vi "Example_Simple Write and Read.vi"() -> ()   [LabVIEW 2018]
uses:
  Types/TCP Config_Cluster.ctl
  MB PLC Client.lvclass
  Types/PLC Config_Cluster.ctl
  Types/MB Ref Range_Cluster.ctl
  Types/Serial Config_Cluster.ctl
  MB PLC Client.lvclass/MB PLC Client.ctl
  791ddaad-21aa-49d1-827f-859499192ae9.vi
  2a8f512b-755f-4b06-8394-ae6f99e928d5.vi
  791ddaad-21aa-49d1-827f-859499192ae9.vi/b864373d-f854-459d-9ae0-25608fa3379f.vi
  Read PLC Config.vi
  2a8f512b-755f-4b06-8394-ae6f99e928d5.vi/835f469a-b32f-4278-a24e-7a39f32541a3.vi
  2a8f512b-755f-4b06-8394-ae6f99e928d5.vi/d20fd42a-0834-430a-aa6f-5ef6bca1fd62.vi
  791ddaad-21aa-49d1-827f-859499192ae9.vi/b864373d-f854-459d-9ae0-25608fa3379f.vi/dbb28a57-791a-4630-bcdd-60eee24abc3a.vi
  791ddaad-21aa-49d1-827f-859499192ae9.vi/b864373d-f854-459d-9ae0-25608fa3379f.vi/66a048c9-f723-4eda-9e66-1b2854b864a8.vi
  2a8f512b-755f-4b06-8394-ae6f99e928d5.vi/835f469a-b32f-4278-a24e-7a39f32541a3.vi/be21e1c6-2a20-46ce-acc9-dfae894bb3c6.vi
  Data/Read from IR DB_byRef.vi
  Data/Read from HR DB_byRef.vi
  Read Data Block.vi
  <vilib>/Utility/error.llb/Error Cluster From Error Code.vi
  Write Holding Registers_Cached.vi
  MB Read_Cached.vi
  Data/MB Data Block.lvclass
  MB PLC Client.lvlib
panel:
  out "error out":errorcluster
  in  "Value2":sgl
  in  "Value1":sgl
  out "Value2":sgl
  out "Value1":sgl
  in  "TCP Config":T1={"IP Address"="localhost", "Port"=502, "Slave ID"=-1, "Timeout"=1000} {"Slave ID" format="%.0x"}
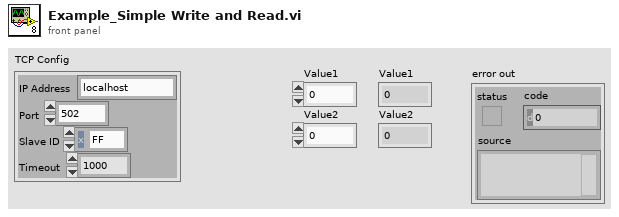
[diagram p1: front panel]
types:
  T1 = typedef "MB PLC Client.lvlib/TCP Config_Cluster.ctl" = cluster{"IP Address":string, "Port":u16, "Slave ID":i8, "Timeout":i32}
  T2 = typedef "MB PLC Client.lvlib/Serial Config_Cluster.ctl" = cluster{"COM Port":string, "Slave ID":u8, "baud rate (bps)":u32, "Mode":enum16{"RTU", "ASCII"}, "Parity":u16, "Flow Control":u16, "Timeout":u32, "Retries":u8, "Stop Bits":u16}
  T3 = typedef "MB PLC Client.lvlib/PLC Config_Cluster.ctl" = cluster{"Use TCP":bool, "Reference Format":u16, "Swap Words":bool, "Poll List":T4[]}
  T4 = typedef "MB PLC Client.lvlib/MB Ref Range_Cluster.ctl" = cluster{"Start":u32, "Qty":u16}
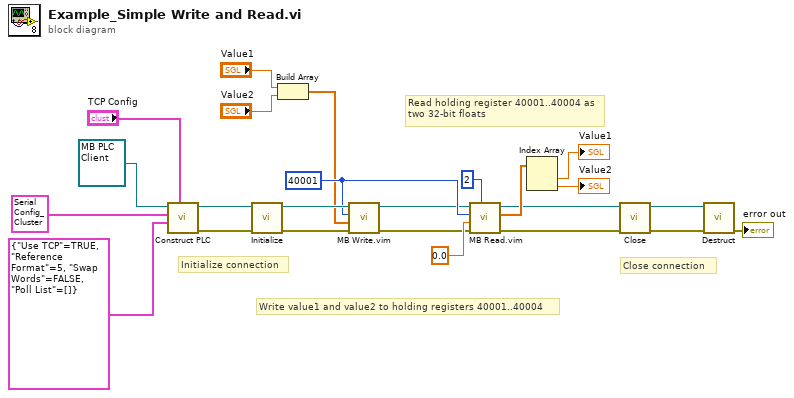
[diagram p0: block diagram]
diagram:
  w12 = u32 40001 ("Modbus Reference")
  # "Close connection"
  # "Write value1 and value2 to holding registers 40001..40004"
  # "Initialize connection"
  # "Read holding register 40001..40004 as\ntwo 32-bit floats"
  n1 = call-dynamic "Construct PLC.vi"("TCP Config"="TCP Config", "PLC Config"=T3 {"Use TCP"=TRUE, "Reference Format"=5, "Swap Words"=FALSE, "Poll List"=[]}, "Serial Config"=T2 {"COM Port"="COM1", "Slave ID"=1, "baud rate (bps)"=460800, "Mode"=enum."RTU", "Parity"=0, "Flow Control"=0, "Timeout"=200, "Retries"=1, "Stop Bits"=10}, "PLC in"=refnum<class "MB PLC Client.lvclass"> refnum) -> ("error out"=w20:errorcluster, "PLC out"=w21:refnum<class "MB PLC Client.lvclass">)  [unwired: 6 in]
  n2 = call-dynamic "Initialize.vi"("error in (no error)"=w20, "PLC in"=w21) -> ("error out"=w11:errorcluster, "PLC out"=w13:refnum<class "MB PLC Client.lvclass">)  [unwired: 8 in]
  n3 = Build Array("Value1", "Value2") -> (w8:sgl[])
  n4 = call "MB Write.vim"("error in (no error)"=w11, "Value"=w8, "Modbus Reference"=w12, "MB PLC in"=w13) -> ("error out"=w6:errorcluster, "MB PLC out"=w7:refnum<class "MB PLC Client.lvclass">)  [unwired: 6 in]
  n5 = call "MB Read.vim"("Quantity (1)"=2, "error in (no error)"=w6, "Type"=sgl 0.0, "Modbus Reference"=w12, "MB PLC in"=w7) -> ("error out"=w4:errorcluster, "Data out"=w18:sgl[], "MB PLC out"=w5:refnum<class "MB PLC Client.lvclass">)  [unwired: 4 in]
  n6 = Index Array(array=w18) -> (element #1=→"Value1":sgl, element #2=→"Value2":sgl)  [unwired: 2 in]
  n7 = call-dynamic "Close.vi"("error in (no error)"=w4, "PLC in"=w5) -> ("error out"=w2:errorcluster, "PLC out"=w3:refnum<class "MB PLC Client.lvclass">)  [unwired: 8 in]
  n8 = call-dynamic "Destruct.vi"("error in (no error)"=w2, "PLC in"=w3) -> ("error out"=→"error out":errorcluster)  [unwired: 9 in]
